vi "Get Last Value from  GIS response.vi"(11 "Command":string) -> (3 "String":string)   [LabVIEW 2022 SP3, in "GIS Printer.lvclass"]
uses:
  GIS Printer.lvclass
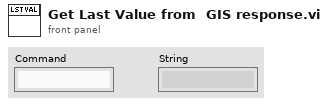
[diagram p1: front panel]
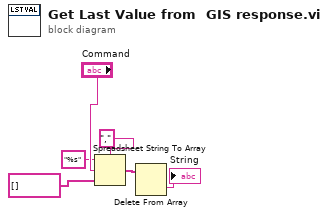
[diagram p0: block diagram]
diagram:
  n1 = Spreadsheet String To Array(delimiter (Tab)="," ("regular expression"), format string="%s", spreadsheet string="Command", array type (2D Dbl)=string[] []) -> (array=w1:string[])
  n2 = Delete From Array(array=w1) -> (deleted portion=→"String":string)  [unwired: 2 in, 1 out]
